vi "Lock In Test.vi"() -> ()   [LabVIEW 2020]
uses:
  Programs/Dependencies/Stanford Research 830/Stanford Research 830.lvlib
panel:
  out "Waveform Graph":sgl[](graph)
  in  "Reset (True)":bool=TRUE
  in  "VISA resource name":refnum<visa-resource-name>
  out "error out":errorcluster
  in  "Maximum Time (10000 ms)":u32=10000
  in  "Number of Points (100)":u32=100
  in  "Channel (1: Channel 1 Display)":u16(ring)=1 items=["Channel 1 Display"=1, "Channel 2 Display"=2]
  in  "Continuous Storage (T: Enable)":bool=TRUE
  in  "Sample Rate (0: 62.5 mHz)":u16(ring) items=["62.5 mHz", "125 mHz", "250 mHz", "500 mHz", "1 Hz", "2 Hz", "4 Hz", "8Hz", "16 Hz", "32 Hz", "64 Hz", "128 Hz", "256 Hz", "512 Hz", "Trigger "]
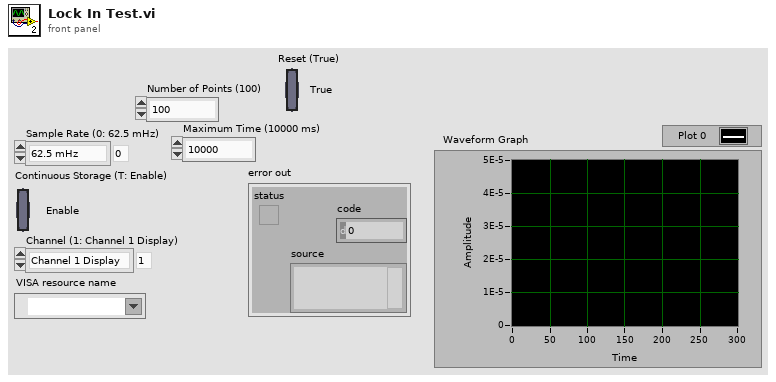
[diagram p1: front panel]
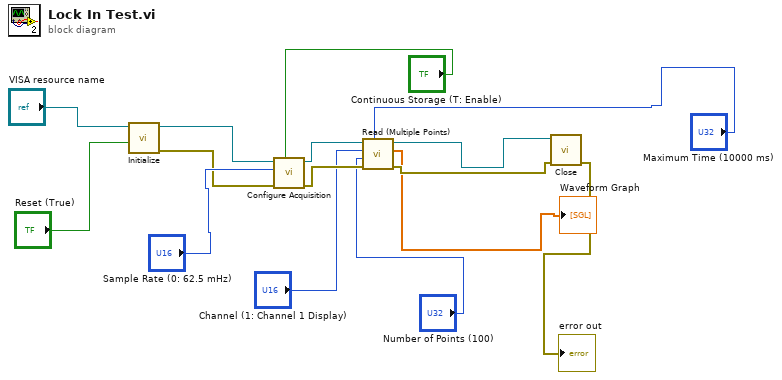
[diagram p0: block diagram]
diagram:
  n1 = call "Initialize.vi"("Reset (True)"="Reset (True)", "VISA resource name"="VISA resource name") -> ("error out"=w4:errorcluster, "VISA resource name out"=w5:refnum<visa-resource-name>)  [unwired: 8 in]
  n2 = call "Configure Acquisition.vi"("Continuous Storage (T: Enable)"="Continuous Storage (T: Enable)", "error in (no error)"=w4, "Sample Rate (0: 62.5 mHz)"="Sample Rate (0: 62.5 mHz)", "VISA resource name"=w5) -> ("error out"=w14:errorcluster, "VISA resource name out"=w15:refnum<visa-resource-name>)  [unwired: 6 in]
  n3 = call "Read (Multiple Points).vi"("Maximum Time (10000 ms)"="Maximum Time (10000 ms)", "error in (no error)"=w14, "Number of Points (100)"="Number of Points (100)", "Channel (1: Channel 1 Display)"="Channel (1: Channel 1 Display)", "VISA resource name"=w15) -> ("error out"=w7:errorcluster, "Measurements"=→"Waveform Graph":sgl[], "VISA resource name out"=w8:refnum<visa-resource-name>)  [unwired: 4 in]
  n4 = call "Close.vi"("error in (no error)"=w7, "VISA resource name"=w8) -> ("error out"=→"error out":errorcluster)  [unwired: 9 in]
